vi "data_LV2.vi"() -> ()   [LabVIEW 2023]
uses:
  Control/Point.ctl
  Control/Points.ctl
  Control/State.ctl
  Control 4.ctl
panel:
  in  "error in (no error)":errorcluster
  in  "Option":T1
  in  "Data":T2
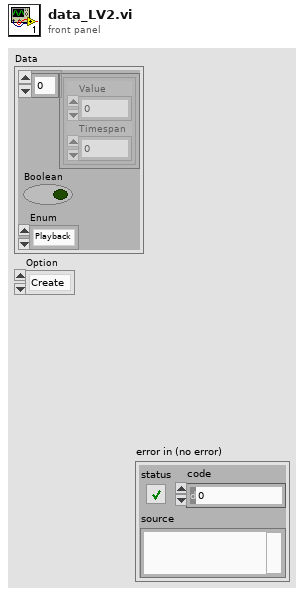
[diagram p1: front panel]
types:
  T1 = typedef "Control 4.ctl" = enum16{"Create", "Gen_ref", "Generate", "Destroy"}
  T2 = typedef "State.ctl" = cluster{T3[], "Boolean":bool, "Enum":T4}
  T3 = typedef "Point.ctl" = cluster{"Value":dbl, "Timespan":dbl}
  T4 = typedef "Points.ctl" = enum16{"Playback", "Record"}
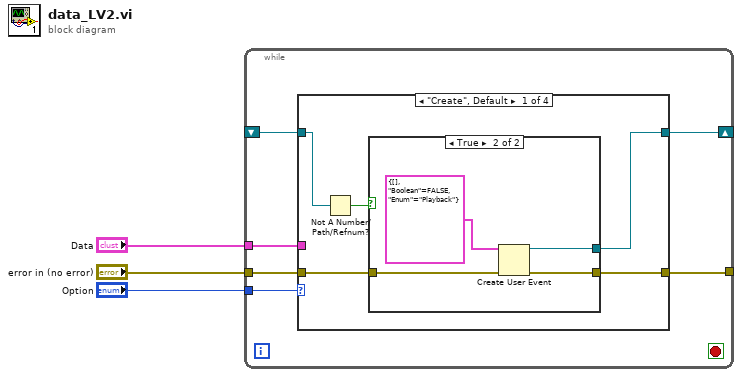
[diagram p0: block diagram]
diagram:
  n1 = while {
    tunnel: "Data" -> [w4]
    shift-right: [w6] -> _
    shift-left: _ -> [w5]
    tunnel: "Option" -> [w9]
    tunnel: "error in (no error)" -> [w8]
    tunnel: [w7] -> _
    stop <- _ stop-if-true
    n2 = case shown="\"Create\", Default" w9 {
      tunnel: w8 -> [w14 _ _ _]
      tunnel: [w13 _ _ _] -> w7
      tunnel: [w12 _ _ _] -> w6
      tunnel: w5 -> [w11 _ _ _]
      tunnel: w4 -> [_ _ _ _]
      frame "Create", Default {
        n3 = Not A Number/Path/Refnum?(number/path/refnum=w11) -> (NaN/Path/Refnum?=w10:bool)
        n4 = case shown="True" w10 {
          tunnel: w14 -> [_ w18]
          tunnel: [_ w17] -> w13
          tunnel: [_ w16] -> w12
          frame False {
          }
          frame True {
            n5 = Create User Event(user event datatype=T2 {[], "Boolean"=FALSE, "Enum"=enum."Playback"} ("Cluster"), error in=w18) -> (user event=w16:refnum<user-event>, error out=w17:errorcluster)
          }
        }
      }
      frame "Gen_ref" {
      }
      frame "Generate" {
      }
      frame "Destroy" {
      }
    }
  }
